vi "01032022 счет квадратный корень.vi"() -> (6 "D":dbl)   [LabVIEW 2020]
panel:
  in  "error in (no error)":errorcluster
  out "x 2":dbl
  out "x1":dbl
  out "D":dbl
  out "x":dbl
  out "String":string
  in  "c":dbl
  in  "b":dbl
  in  "a":dbl
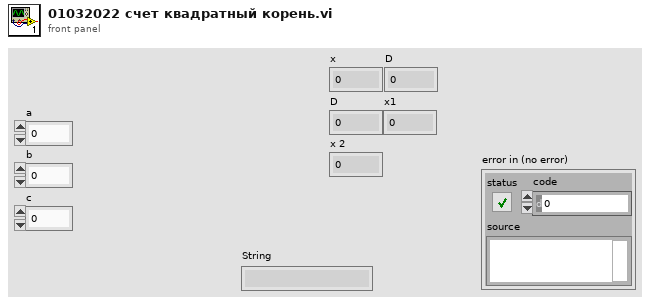
[diagram p1: front panel]
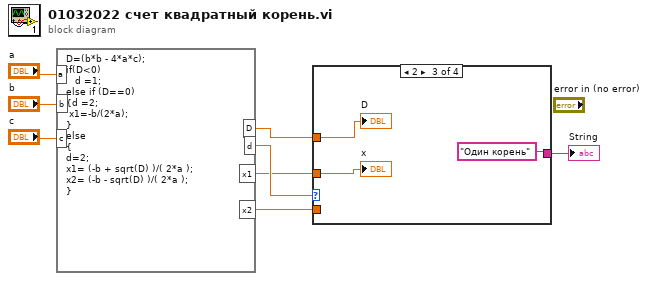
[diagram p0: block diagram]
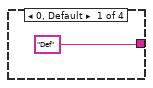
[diagram p2: hidden frame]
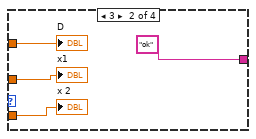
[diagram p3: hidden frame]
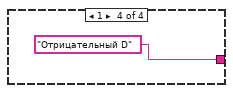
[diagram p4: hidden frame]
diagram:
  n1 = formula code="D=(b*b - 4*a*c);\nif(D<0)\n   d =1;\nelse if (D==0)\n{d =2;\n x1=-b/(2*a);\n}\nelse \n{\nd=2;\nx1= (-b + sqrt(D) )/( 2*a );\nx2= (-b - sqrt(D) )/( 2*a );\n}"("a"="a", "b"="b", "c"="c") -> ("D"=w5:dbl, "d"=w4:dbl, "x1"=w2:dbl, "x2"=w1:dbl)
  n2 = case shown="2" w4 {
    tunnel: w5 -> [_ w13 w16 _]
    tunnel: ["Def" "ok" "Один корень" "Отрицательный D"] -> w3
    tunnel: w2 -> [_ w12 w15 _]
    tunnel: w1 -> [_ w11 _ _]
    frame 0, Default {
    }
    frame 3 {
      "D" <- w13
      "x1" <- w12
      "x 2" <- w11
    }
    frame 2 {
      "D" <- w16
      "x" <- w15
    }
    frame 1 {
    }
  }
  "String" <- w3
